vi "VariantToSimpleCluster.vi"(8 "error in (no error)":errorcluster, 11 "Variant":variant) -> (0 "error out":errorcluster, 2 "SimpleCluster":T1 {"Single" format="%#.19f"}, 3 "Variant (dup)":variant)   [LabVIEW 2015, in "MsgPack.lvlib"]
uses:
  MsgPack.lvlib
  Simple Cluster.ctl
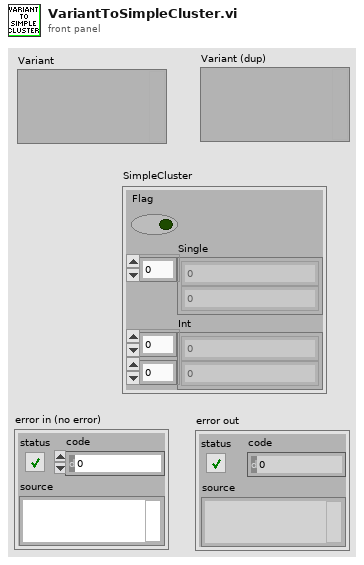
[diagram p1: front panel]
types:
  T1 = typedef "MsgPack.lvlib/Simple Cluster.ctl" = cluster{"Flag":bool, "Single":sgl[], "Int":i32[][]}
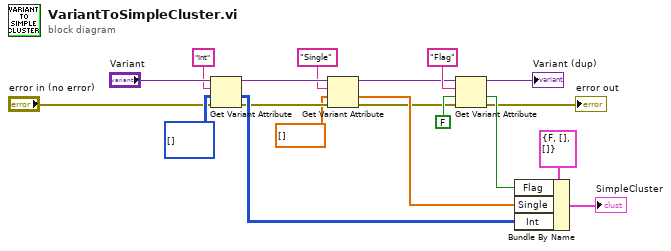
[diagram p0: block diagram]
diagram:
  n1 = Get Variant Attribute(Variant="Variant", name="Int", default value (empty Variant)=i32[][] [], error in="error in (no error)") -> (duplicate Variant=w13:variant, value=w15:i32[][], error out=w14:errorcluster)  [unwired: 1 out]
  n2 = Get Variant Attribute(Variant=w13, name="Single", default value (empty Variant)=sgl[] [], error in=w14) -> (duplicate Variant=w7:variant, value=w17:sgl[], error out=w8:errorcluster)  [unwired: 1 out]
  n3 = Get Variant Attribute(Variant=w7, name="Flag", default value (empty Variant)=FALSE, error in=w8) -> (duplicate Variant=→"Variant (dup)":variant, value=w16:bool, error out=→"error out":errorcluster)  [unwired: 1 out]
  n4 = Bundle By Name(cluster=T1 {"Flag"=FALSE, "Single"=[], "Int"=[]} ("Packet"), "Flag"=w16, "Single"=w17, "Int"=w15) -> (→"SimpleCluster":T1)
